vi "HRM-init-select_hardware.vi"(8 "error in (no error)":errorcluster) -> (0 "error out":errorcluster, 2 "Hardware type out":T1)   [LabVIEW 2020]
uses:
  HRM-init-hardware_selector.ctl
panel:
  in  "Cancel Button":bool
  in  "OK Button":bool
  in  "Hardware type":T1
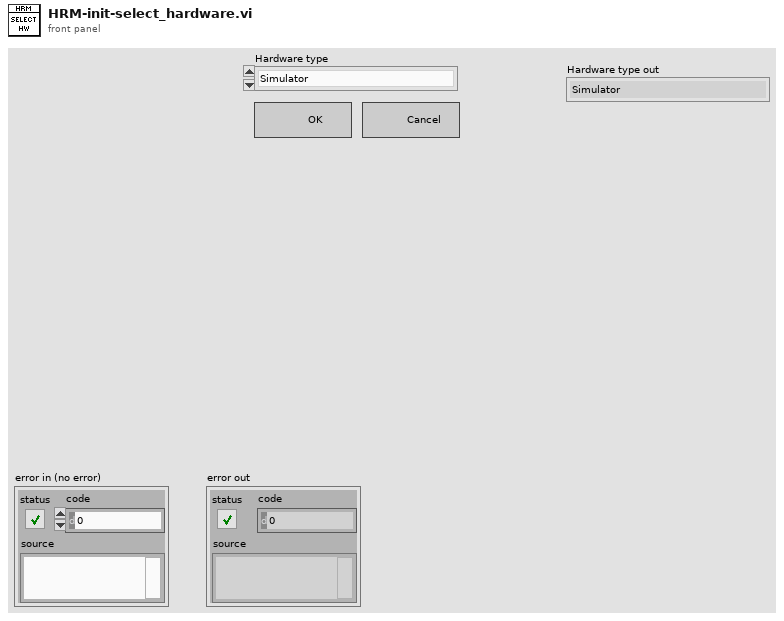
[diagram p1: front panel]
types:
  T1 = typedef "HRM-init-hardware_selector.ctl" = enum16{"Simulator", "myDAQ", "Arduino", "Analog Discovery"}
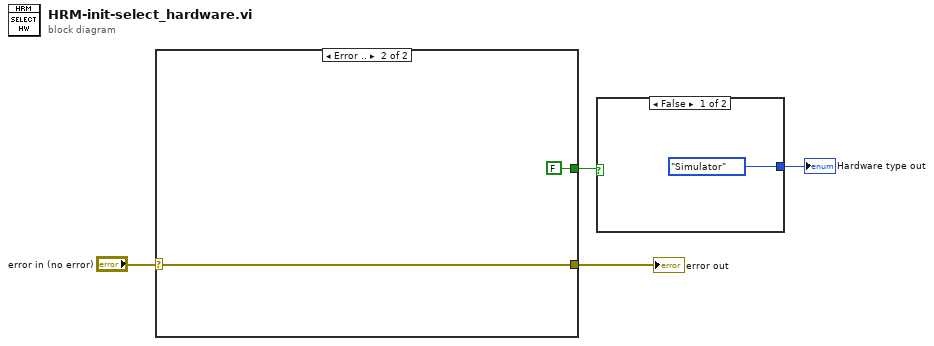
[diagram p0: block diagram]
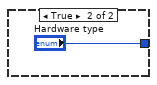
[diagram p2: hidden frame]
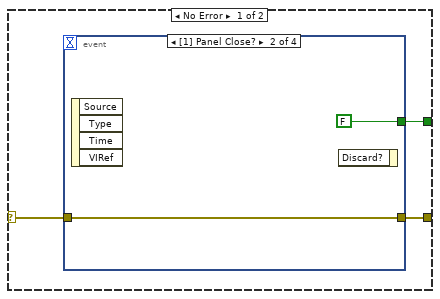
[diagram p3: hidden frame]
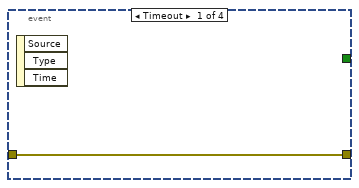
[diagram p4: hidden frame]
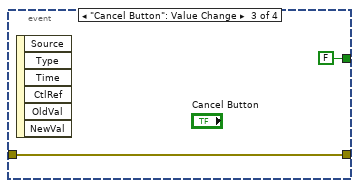
[diagram p5: hidden frame]
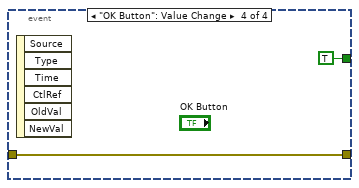
[diagram p6: hidden frame]
diagram:
  n1 = case shown="Error .." "error in (no error)" {
    selector: "error in (no error)" -> [w7 w16]
    tunnel: [w6 w16] -> w3
    tunnel: [w5 FALSE] -> w2
    frame No Error {
      n2 = event shown="[1] Panel Close?" {
        selector: _ -> [_ _ _ _]
        dyn-events: _ -> [_ _ _ _]
        timeout: _ -> [_ _ _ _]
        tunnel: w7 -> [w8 w9 w12 w14]
        tunnel: [w8 w9 w12 w14] -> w6
        tunnel: [_ FALSE FALSE TRUE] -> w5
        event Timeout {
          n3 = event-data() -> ()  [unwired: 1 in, 3 out]
        }
        event Panel Close? {
          n4 = event-data() -> ()  [unwired: 1 in, 4 out]
          n5 = event-data() -> ()  [unwired: 2 in, 1 out]
        }
        event "Cancel Button": Value Change {
          n6 = event-data() -> ()  [unwired: 1 in, 6 out]
        }
        event "OK Button": Value Change {
          n7 = event-data() -> ()  [unwired: 1 in, 6 out]
        }
      }
    }
    frame Error {
    }
  }
  "error out" <- w3
  n8 = case shown="False" w2 {
    tunnel: [HRM-init-hardware_selector."Simulator" ("Hardware type 2") "Hardware type"] -> w1
    frame False {
    }
    frame True {
    }
  }
  "Hardware type out" <- w1
